vi "Write permission.vi"(8 "error in (no error)":errorcluster, 10 "permission":T1=enum."User", 11 "Person in":refnum<class "Person.lvclass">) -> (0 "error out":errorcluster, 3 "Person out":refnum<class "Person.lvclass">)   [LabVIEW 2014, in "Person.lvclass"]
uses:
  Person.lvclass
  DEF-Permission.ctl
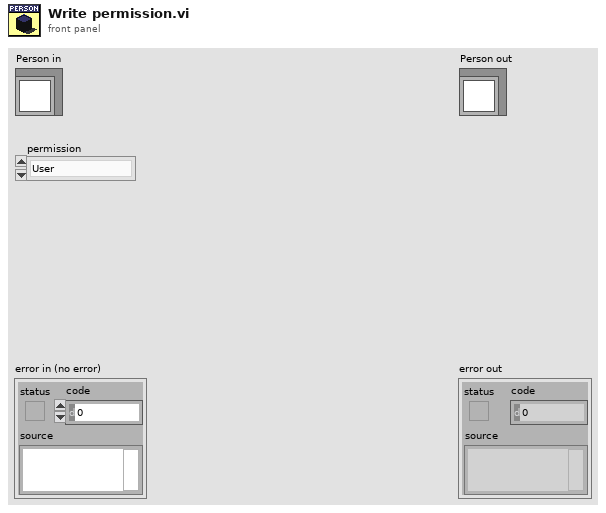
[diagram p1: front panel]
types:
  T1 = typedef "Person.lvclass/DEF-Permission.ctl" = enum16{"Visitor", "User", "Admin"}
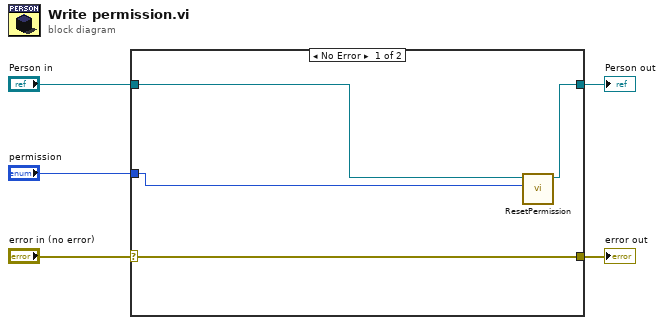
[diagram p0: block diagram]
diagram:
  n1 = case shown="No Error" "error in (no error)" {
    selector: "error in (no error)" -> [w9 w10]
    tunnel: [w9 w10] -> w4
    tunnel: [w6 w11] -> w2
    tunnel: "Person in" -> [w8 w11]
    tunnel: "permission" -> [w7 _]
    frame No Error {
      n2 = call "ResetPermission.vi"("permission"=w7, "Person in"=w8) -> ("Person out"=w6:refnum<class "Person.lvclass">)  [unwired: 8 in, 1 out]
    }
    frame Error {
    }
  }
  "error out" <- w4
  "Person out" <- w2
